vi "G#ModifyAttributeDiagramTemplate.vi"   [LabVIEW 2017]
doc: "This is a G# modify attribute DVR structure. Paste this in your diagram together with the GetAttributes to modify the attributes."
types:
  T1 = typedef "G#Template.lvclass/ObjectAttributes.ctl" = cluster{"Numeric":dbl}
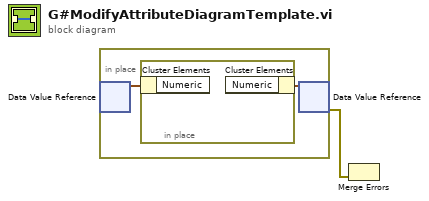
[diagram p0: block diagram]
diagram:
  n1 = in-place {
    n2 = in-place-dvr #1() -> (w2:T1)  [unwired: 1 in, 1 out]
    n3 = in-place {
      n4 = in-place-cluster #2(w2) -> ()  [unwired: 1 out]
      n5 = in-place-cluster #2() -> (w3:T1)  [unwired: 1 in]
    }
    n6 = in-place-dvr #1(w3) -> (w1:errorcluster)  [unwired: 1 out]
  }
  n7 = Merge Errors(w1) -> ()  [unwired: 1 in, 1 out]
